vi "Initialize.vi"(8 "update":refnum<k4>, 11 "TagData in":refnum<class "TagData.lvclass">) -> (3 "TagData out":refnum<class "TagData.lvclass">)   [LabVIEW 2020, in "Tag-str.lvlib" / "TagData.lvclass"]
uses:
  <extravilib>/ChannelInstances/Tag-str/TagData.lvclass
  <extravilib>/ChannelInstances/Tag-str/TagData.lvclass/TagData.ctl
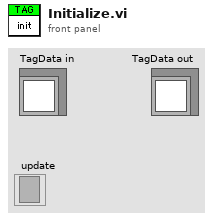
[diagram p1: front panel]
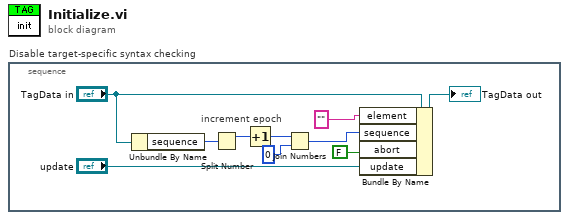
[diagram p0: block diagram]
diagram:
  n1 = stacked-sequence "Disable target-specific syntax checking" {
    frame #0 {
      # "increment epoch"
      n2 = Unbundle By Name("TagData in") -> ("sequence"=w6:u64)
      n3 = Split Number(x=w6) -> (hi(x)=w5:u32)  [unwired: 1 out]
      n4 = Increment(x=w5) -> (x+1=w4:u32)
      n5 = Join Numbers(hi=w4, lo=u32 0 ("lo(x)")) -> ((hi.lo)=w2:u64)
      n6 = Bundle By Name(cluster="TagData in", "element"="", "sequence"=w2, "abort"=FALSE, "update"="update") -> (→"TagData out":refnum<class "TagData.lvclass">)
    }
  }
